vi "Save Fake Flag.vi"(6 "section":string, 7 "error in (no error)":errorcluster, 9 "Fake":bool, 10 "config ref in":T1) -> (0 "error out":errorcluster, 3 "config ref out":T1)   [LabVIEW 2013]
uses:
  <vilib>/Utility/config.llb/Config Data RefNum.ctl
  <vilib>/Utility/config.llb/Write Key (Boolean).vi
  <vilib>/Utility/config.llb/NI_LVConfig.lvlib
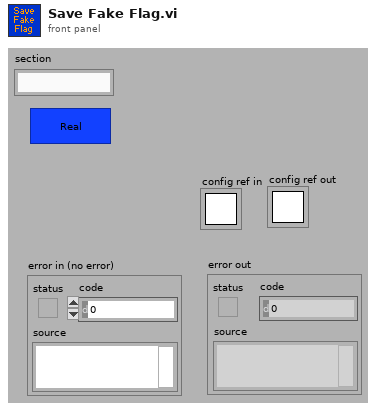
[diagram p1: front panel]
types:
  T1 = typedef "NI_LVConfig.lvlib/Config Data RefNum.ctl" = refnum<k1>
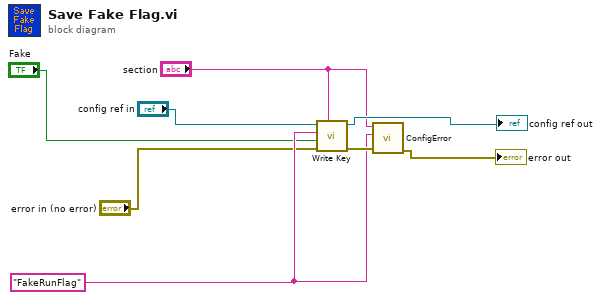
[diagram p0: block diagram]
diagram:
  w4 = "FakeRunFlag" ("key")
  n1 = call-poly <vilib>:"Write Key.vi"("section"="section", "error in (no error)"="error in (no error)", "value"="Fake", "key"=w4, "refnum"="config ref in") -> ("error out"=w8:errorcluster, "refnum out"=→"config ref out":T1)  [unwired: 4 in, 1 out]
  n2 = call "ConfigError.vi"("error in (no error)"=w8, "Key"=w4, "Section"="section") -> ("error out"=→"error out":errorcluster)  [unwired: 8 in]
